vi "扭矩计算公式.vi"(1 "电机ID":string, 2 "扭矩":dbl(slide) scale=-12.0..12.0) -> (0 "最终输出报文 2":string)   [LabVIEW 2023]
panel:
  out "十六进制整型字符串":string
  in  "选项卡控件":enum32{"选项卡 1", "选项卡 2"}(tab)
  out "最终输出报文":string
  out "未左移前字符串":string
  out "扭矩转换所得数值":u16
  in  "输入字符串":string="AT\u0007è\f\b\u0005p\u0000\u0000\u0001\u0000\u0000\u0000\r\n"
  in  "通信模式":string="01"
  out "替换子字符串":string
  out "连接为字符串":string
  out "16进制转换":string
  out "16进制转换10进制":u32
  out "二进制转换":string
  out "左移3位加100":string
  out "检验转为16进制":string
  out "十进制数":i32
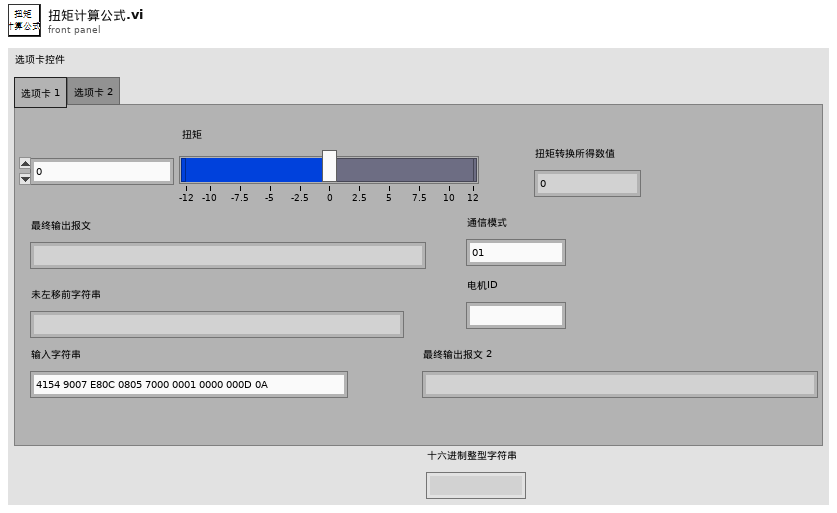
[diagram p1: front panel]
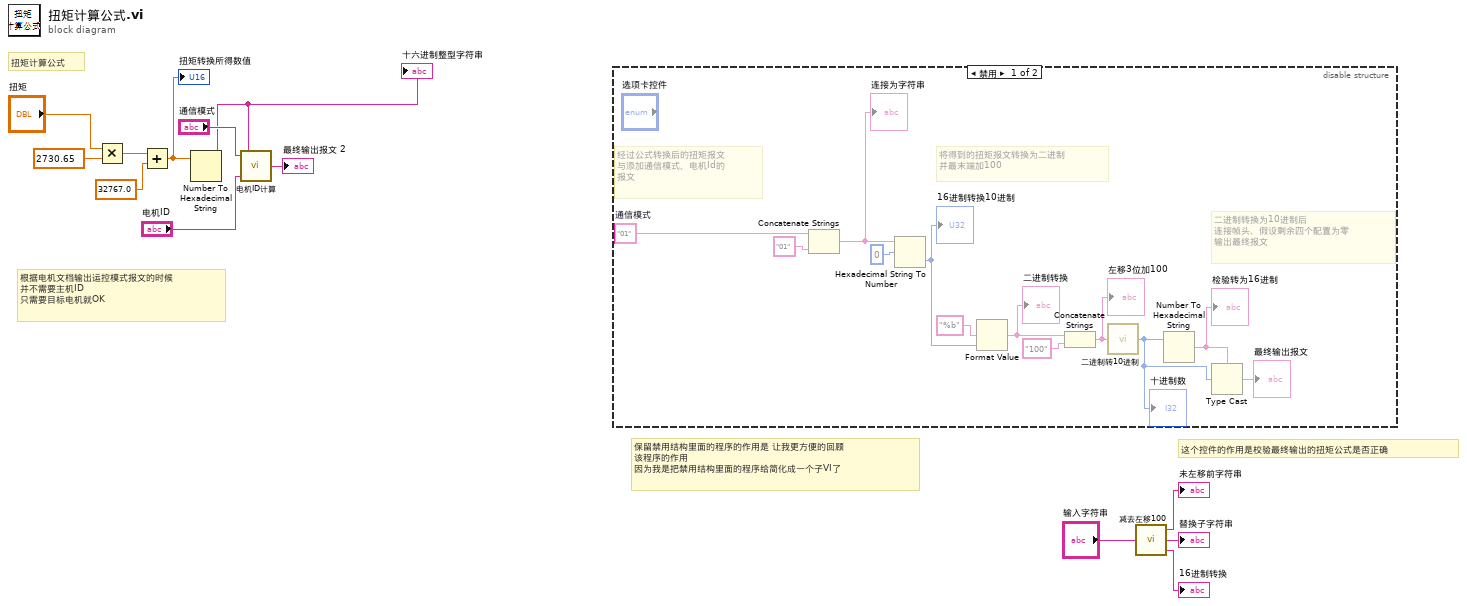
[diagram p0: block diagram]
diagram:
  # "根据电机文档输出运控模式报文的时候\n并不需要主机ID\n只需要目标电机就OK"
  # "保留禁用结构里面的程序的作用是 让我更方便的回顾 \n该程序的作用 \n因为我是把禁用结构里面的程序给简化成一个子VI了"
  # "这个控件的作用是校验最终输出的扭矩公式是否正确"
  # "扭矩计算公式"
  n1 = Multiply(x="扭矩", y=2730.65) -> (x*y=w11:dbl)
  n2 = Add(x=w11, y=32767.0) -> (x+y=w9:dbl)
  "扭矩转换所得数值" <- w9
  n3 = Number To Hexadecimal String(2:w9) -> (0:w1:string)  [unwired: 1 in]
  "十六进制整型字符串" <- w1
  n4 = call "电机ID计算.vi"("电机ID"="电机ID", "主机id"=w1, "通信模式"="通信模式") -> ("最终输出报文"=→"最终输出报文 2":string)
  n5 = disable-structure shown="禁用" {
    frame Disabled {
      w26 = "01"  # 通信模式
      # "二进制转换为10进制后\n连接帧头、假设剩余四个配置为零\n输出最终报文"
      # "将得到的扭矩报文转换为二进制\n并最末端加100"
      # "经过公式转换后的扭矩报文\n与添加通信模式、电机Id的\n报文"
      n6 = Concatenate Strings(w26, "01" ("字符串")) -> (w17:string, w14:string)
      "连接为字符串" <- w17
      n7 = Hexadecimal String To Number(string=w17, offset=0 ("偏移量")) -> (number=w18:u32)  [unwired: 1 in, 1 out]
      "16进制转换10进制" <- w18
      n8 = Format Value(format string="%b" ("格式字符串"), value (0)=w18) -> (output string=w21:string)  [unwired: 1 in]
      "二进制转换" <- w21
      n9 = Concatenate Strings(w21, "100" ("字符串")) -> (w20:string)
      "左移3位加100" <- w20
      n10 = call "二进制转10进制.vi"("字符串"=w20) -> ("十进制数"=w24:i32)
      "十进制数" <- w24
      n11 = Number To Hexadecimal String(2:w24) -> (0:w23:string)  [unwired: 1 in]
      "检验转为16进制" <- w23
      n12 = Type Cast(type=w23, x=w24) -> (*(type *) &x=→"最终输出报文":string)
    }
    frame Enabled {
    }
  }
  n13 = call "减去左移100.vi"("输入字符串"="输入字符串") -> ("结果字符串"=→"未左移前字符串":string, "替换子字符串"=→"替换子字符串":string, "16进制转换"=→"16进制转换":string)
